vi "getBuildWorkerDefaultConfiguration.vi"(8 "error in (no error)":errorcluster, 10 "configuration file path":path, 11 "BuildWorker Basics in":refnum<class "BuildWorker Local.lvclass">) -> (0 "error out":errorcluster, 2 "#Max Worker":i32, 3 "BuildWorker Basics out":refnum<class "BuildWorker Local.lvclass">)   [LabVIEW 2017, in "BuildWorker Interface.lvlib" / "BuildWorker Local.lvclass"]
uses:
  BuildWorker Local.lvclass
  BuildWorker/BuildWorker.lvclass
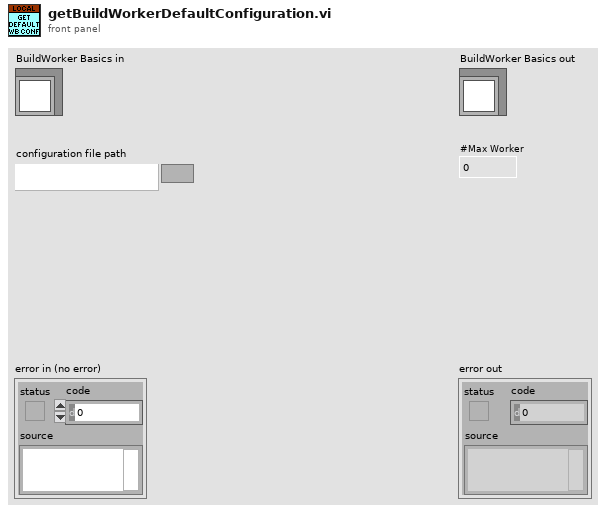
[diagram p1: front panel]
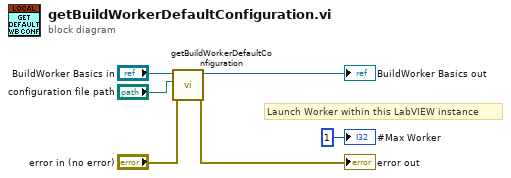
[diagram p0: block diagram]
diagram:
  # "Launch Worker within this LabVIEW instance"
  n1 = call-parent "getBuildWorkerDefaultConfiguration.vi"("error in (no error)"="error in (no error)", "configuration file path"="configuration file path", "BuildWorker in"="BuildWorker Basics in") -> ("error out"=→"error out":errorcluster, "BuildWorker out"=→"BuildWorker Basics out":refnum<class "BuildWorker Local.lvclass">)  [unwired: 6 in, 1 out]
  "#Max Worker" <- 1 ("#Max Worker")
